vi "oTp.vi"() -> ()   [LabVIEW 2025]
panel:
  out "OTP":dbl
  in  "stop":bool
  in  "PUSH BUTTON":bool
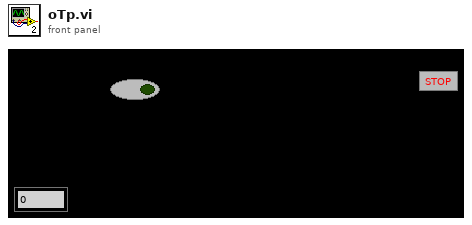
[diagram p1: front panel]
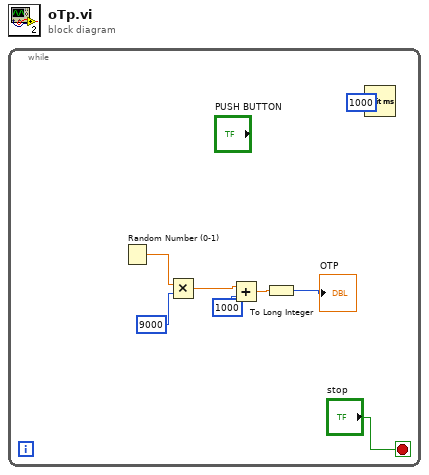
[diagram p0: block diagram]
diagram:
  n1 = while {
    stop <- "stop" stop-if-true
    n2 = Random Number (0-1)() -> (number: 0 to 1=w7:dbl)
    n3 = Multiply(x=w7, y=9000) -> (x*y=w6:dbl)
    n4 = Add(x=w6, y=1000) -> (x+y=w2:dbl)
    n5 = To Long Integer(number=w2) -> (32bit integer=→"OTP":i32)
    n6 = Wait (ms)(milliseconds to wait=1000) -> ()  [unwired: 1 out]
  }
